vi "quadratic equation solver.vi"() -> ()   [LabVIEW 2024]
panel:
  out "conditions":string
  out "root  2":dbl
  out "root 1":dbl
  in  "c":dbl
  in  "b":dbl
  in  "a":dbl
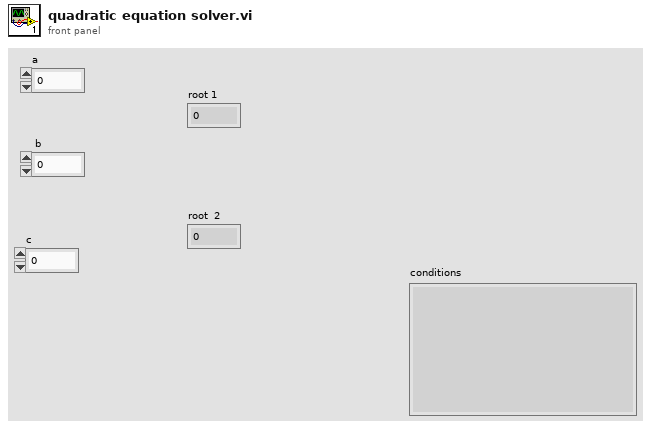
[diagram p1: front panel]
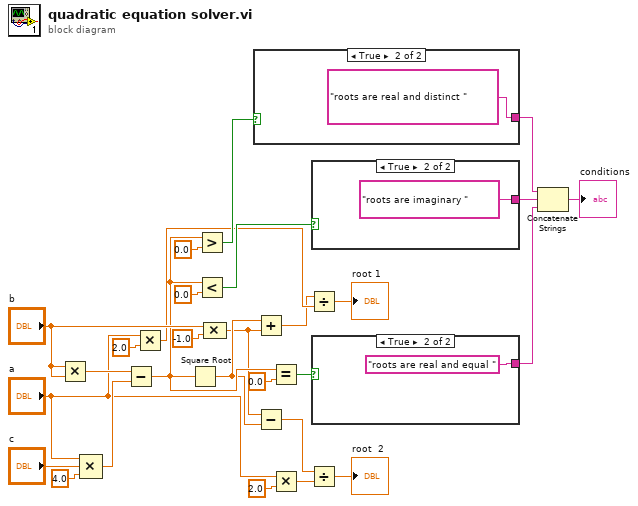
[diagram p0: block diagram]
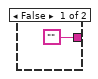
[diagram p2: hidden frame]
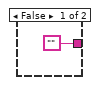
[diagram p3: hidden frame]
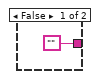
[diagram p4: hidden frame]
diagram:
  n1 = Multiply(x="b", y="b") -> (x*y=w25:dbl)
  n2 = Compound Arithmetic op=MULTIPLY("a", "c", 4.0 ("value")) -> (w27:dbl)
  n3 = Subtract(x=w25, y=w27) -> (x-y=w14:dbl)
  n4 = Multiply(x="a", y=2.0) -> (x*y=w9:dbl)
  n5 = Square Root(x=w14) -> (sqrt(x)=w2:dbl)
  n6 = Greater?(x=w14, y=0.0) -> (0:w22:bool)
  n7 = Less?(x=w14, y=0.0) -> (x < y?=w21:bool)
  n8 = Compound Arithmetic op=MULTIPLY("b", -1.0 ("value")) -> (w1:dbl)
  n9 = case shown="True" w22 {
    tunnel: ["" "roots are real and distinct "] -> w5
    frame False {
    }
    frame True {
    }
  }
  n10 = Add(x=w2, y=w1) -> (x+y=w8:dbl)
  n11 = Subtract(x=w1, y=w2) -> (x-y=w7:dbl)
  n12 = Equal?(x=w14, y=0.0) -> (x = y?=w20:bool)
  n13 = Multiply(x="a", y=2.0) -> (x*y=w10:dbl)
  n14 = Divide(x=w8, y=w9) -> (x/y=→"root 1":dbl)
  n15 = Divide(x=w7, y=w10) -> (x/y=→"root  2":dbl)
  n16 = case shown="True" w21 {
    tunnel: ["" "roots are imaginary "] -> w4
    frame False {
    }
    frame True {
    }
  }
  n17 = case shown="True" w20 {
    tunnel: ["" "roots are real and equal "] -> w3
    frame False {
    }
    frame True {
    }
  }
  n18 = Concatenate Strings(w5, w4, w3) -> (→"conditions":string)
